vi "ENCODER-READ.vi"(8 "error in (no error)":errorcluster, 11 "ARRAY IN":string[](array[string])) -> (0 "error out":errorcluster, 2 "VALOR ENCODER":u16)   [LabVIEW 2014, in "CAP-USB.lvlib"]
doc: "Se encarga de la lectura de los valores del encoder enviados \npor el CAP-USB"
uses:
  CAP-USB.lvlib
  0-Nivel/Enum DI-Reader.ctl
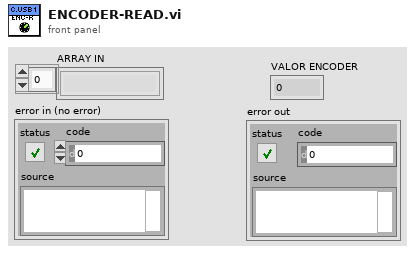
[diagram p1: front panel]
types:
  T1 = typedef "CAP-USB.lvlib/Enum DI-Reader.ctl" = enum16{"IDLE", "Detect XX", "Detect YY", "Valor", ""}
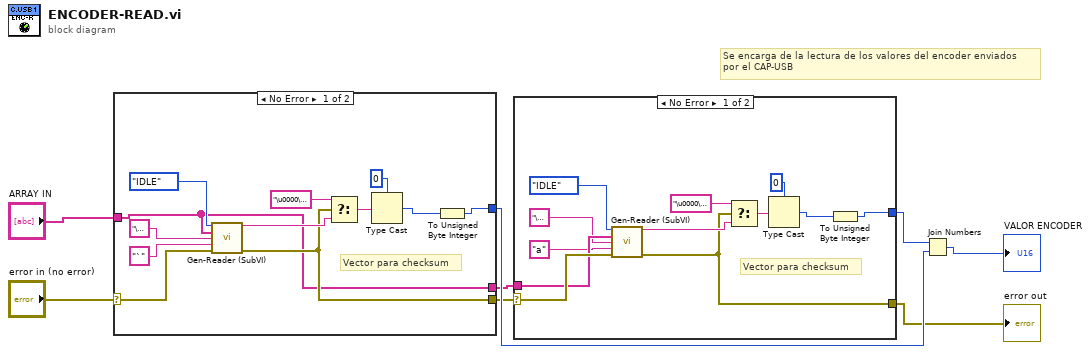
[diagram p0: block diagram]
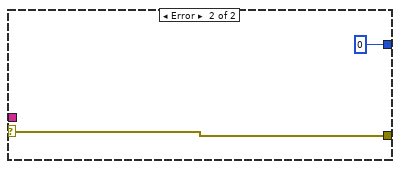
[diagram p2: hidden frame]
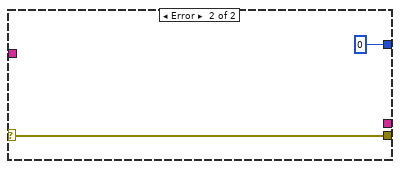
[diagram p3: hidden frame]
diagram:
  # "Se encarga de la lectura de los valores del encoder enviados \npor el CAP-USB"
  n1 = case shown="No Error" "error in (no error)" {
    selector: "error in (no error)" -> [w17 w22]
    tunnel: [w18 w22] -> w2
    tunnel: [w9 u8 0 ("default (0 U32)")] -> w4
    tunnel: "ARRAY IN" -> [w13 _]
    tunnel: [w13 _] -> w3
    frame No Error {
      # "Vector para checksum"
      n2 = call "Gen-Reader (SubVI).vi"("Enum"=Enum_DI-Reader."IDLE", "ARRAY IN"=w13, "XX"="\u0003", "YY"="`", "error in (no error)"=w17) -> ("read buffer"=w20:string, "error out"=w18:errorcluster)  [unwired: 8 in, 1 out]
      n3 = Select(t="\u0000\u0000", s=w18, f=w20) -> (s? t:f=w16:string)
      n4 = Type Cast(type=u8 0 ("default (0 U32)"), x=w16) -> (*(type *) &x=w10:u8)
      n5 = To Unsigned Byte Integer(number=w10) -> (unsigned 8bit integer=w9:u8)
    }
    frame Error {
    }
  }
  n6 = case shown="No Error" w2 {
    selector: w2 -> [w31 w36]
    tunnel: [w32 w36] -> w1
    tunnel: [w23 u8 0 ("default (0 U32)")] -> w5
    tunnel: w3 -> [w27 _]
    frame No Error {
      # "Vector para checksum"
      n7 = call "Gen-Reader (SubVI).vi"("Enum"=Enum_DI-Reader."IDLE", "ARRAY IN"=w27, "XX"="\u0003", "YY"="a", "error in (no error)"=w31) -> ("read buffer"=w34:string, "error out"=w32:errorcluster)  [unwired: 8 in, 1 out]
      n8 = Select(t="\u0000\u0000", s=w32, f=w34) -> (s? t:f=w30:string)
      n9 = Type Cast(type=u8 0 ("default (0 U32)"), x=w30) -> (*(type *) &x=w24:u8)
      n10 = To Unsigned Byte Integer(number=w24) -> (unsigned 8bit integer=w23:u8)
    }
    frame Error {
    }
  }
  "error out" <- w1
  n11 = Join Numbers(hi=w5, lo=w4) -> ((hi.lo)=→"VALOR ENCODER":u16)
